vi "Autonomus.vi"(11 "RobotData":T1) -> ()   [LabVIEW 2019, in "Robot.lvlib" / "Panzer.lvclass"]
uses:
  Panzer.lvclass
  TypeDefs/RobotObjects.ctl
  Drive/Tank Drive/Tank Drive.lvclass
  Pnematics control/Pneumatics.lvclass
  Vision/Vision.lvclass
  Joysticks/Joysticks.lvclass
  Elevator/Elevator.lvclass
  Hatch/Hatch.lvclass
  Cargo/Cargo.lvclass
  DriveOld/Drive.lvclass
  Robot.lvclass
  Control Panel/Control Panel.lvclass
  Climber/Climber.lvclass
  Turret/Turret.lvclass
  PowerCellHandler/Power Cell Handler.lvclass
  Robot.lvclass/Robot.ctl
  PowerCellHandler/Controls/Shooting Position.ctl
  Data Members/Read Waits.vi
  Pnematics control/Solenoids/Solenoids.lvclass
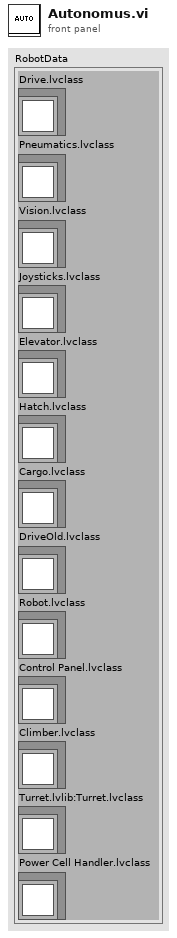
[diagram p1: front panel]
types:
  T1 = typedef "RobotObjects.ctl" = cluster{"Drive.lvclass":refnum<class "Tank Drive.lvclass">, "Pneumatics.lvclass":refnum<class "Pneumatics.lvclass">, "Vision.lvclass":refnum<class "Vision.lvclass">, "Joysticks.lvclass":refnum<class "Joysticks.lvclass">, "Elevator.lvclass":refnum<class "Elevator.lvclass">, "Hatch.lvclass":refnum<class "Hatch.lvclass">, "Cargo.lvclass":refnum<class "Cargo.lvclass">, "DriveOld.lvclass":refnum<class "Drive.lvclass">, "Robot.lvclass":refnum<class "Robot.lvclass">, "Control Panel.lvclass":refnum<class "Control Panel.lvclass">, "Climber.lvclass":refnum<class "Climber.lvclass">, "Turret.lvlib:Turret.lvclass":refnum<class "Turret.lvclass">, "Power Cell Handler.lvclass":refnum<class "Power Cell Handler.lvclass">}
  T2 = cluster{"Wait Before Shoot":dbl, "Wait Before Drive":dbl}
  T3 = typedef "Power Cell Handler.lvlib/Power Cell Handler.lvclass/Shooting Position.ctl" = enum16{"Rest", "Front", "Middle", "Back"}
  T4 = typedef "Pneumatics control.lvlib/Pneumatics.lvclass/Solenoids.ctl" = cluster{"Air Cooler":refnum<class "Solenoids.lvclass">, "ArmLock":refnum<class "Solenoids.lvclass">, "HatchArm":refnum<class "Solenoids.lvclass">, "HatchGrabber":refnum<class "Solenoids.lvclass">, "CPDeploy":refnum<class "Solenoids.lvclass">, "Power Cells Intake":refnum<class "Solenoids.lvclass">}
  T5 = typedef "Turret.lvlib/Turret.lvclass/Turret control states.ctl" = enum16{"Position", "Offset", "IMU"}
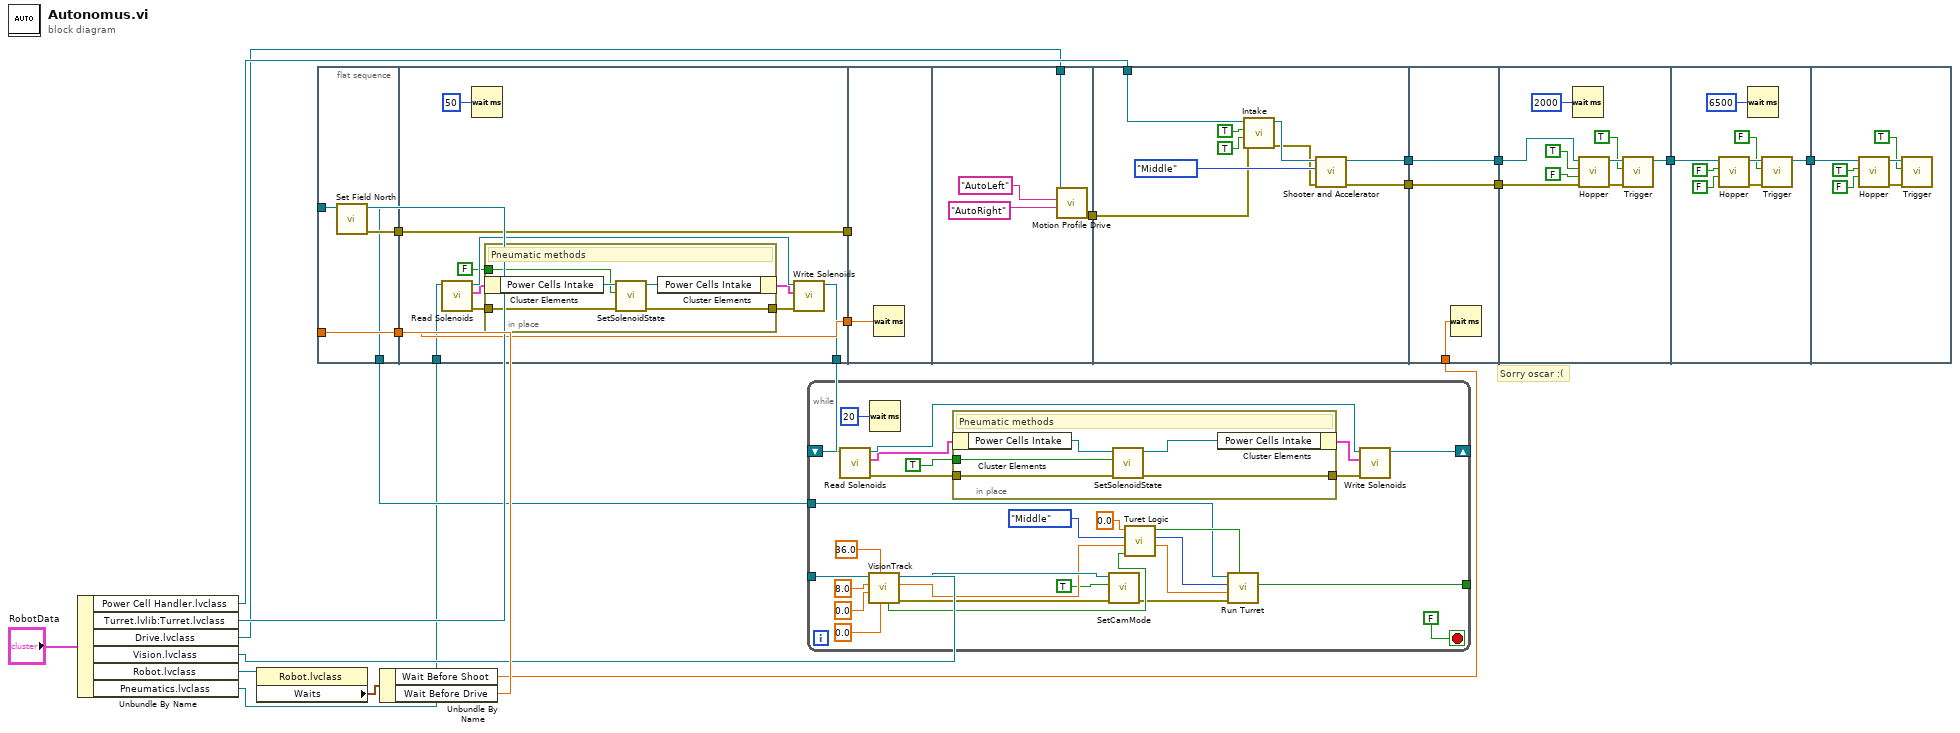
[diagram p0: block diagram]
diagram:
  # "Sorry oscar :("
  n1 = Unbundle By Name("RobotData") -> ("Power Cell Handler.lvclass"=w15:refnum<class "Power Cell Handler.lvclass">, "Turret.lvlib:Turret.lvclass"=w19:refnum<class "Turret.lvclass">, "Drive.lvclass"=w2:refnum<class "Tank Drive.lvclass">, "Vision.lvclass"=w17:refnum<class "Vision.lvclass">, "Robot.lvclass"=w22:refnum<class "Robot.lvclass">, "Pneumatics.lvclass"=w6:refnum<class "Pneumatics.lvclass">)
  n2 = property class="Robot.lvclass"(reference=w22) -> ("Waits"=w21:T2)  [unwired: 1 in, 2 out]
  n3 = flat-sequence {
    tunnel: w20 -> [w27]
    tunnel: [w25] -> w10
    tunnel: [w27] -> w8
    tunnel: w19 -> [w26]
    tunnel: [w24] -> w16
    tunnel: w10 -> [w38]
    tunnel: [w38] -> w9
    tunnel: w8 -> [w37]
    tunnel: [w37] -> w7
    tunnel: w6 -> [w29]
    tunnel: [w28] -> w5
    tunnel: w9 -> [_]
    tunnel: w7 -> [w44]
    tunnel: w2 -> [w46]
    tunnel: [w45] -> w1
    tunnel: w15 -> [w53]
    tunnel: [w56] -> w13
    tunnel: [w55] -> w12
    tunnel: w1 -> [w50]
    tunnel: w18 -> [w60]
    tunnel: [w59] -> w14
    tunnel: w13 -> [w59]
    tunnel: w12 -> [w58]
    tunnel: [w58] -> w11
    tunnel: w14 -> [w66]
    tunnel: w11 -> [w65]
    tunnel: [w61] -> w4
    tunnel: w4 -> [w72]
    tunnel: [w70] -> w3
    tunnel: w3 -> [w78]
    frame #0 {
      n4 = call "Set Field North.vi"("Turret in"=w26) -> ("error out"=w25:errorcluster, "Turret out"=w24:refnum<class "Turret.lvclass">)  [unwired: 9 in]
    }
    frame #1 {
      n5 = call-dynamic "Read Solenoids.vi"("Pneumatics in"=w29) -> ("error out"=w34:errorcluster, "Solenoids"=w35:T4, "Pneumatics out"=w36:refnum<class "Pneumatics.lvclass">)  [unwired: 8 in]
      n6 = Wait (ms)(milliseconds to wait=u32 50) -> ()  [unwired: 1 out]
      n7 = in-place {
        in-place-border: w34 -> [w42]
        in-place-border: [w40] -> w32
        in-place-border: FALSE ("f") -> [w39]
        # "Pneumatic methods"
        n8 = in-place-cluster #1(w35) -> ("Power Cells Intake"=w41:refnum<class "Solenoids.lvclass">)
        n9 = call-dynamic "SetSolenoidState.vi"("error in (no error)"=w42, "Solenoid On?"=w39, "Solenoids in"=w41) -> ("error out"=w40:errorcluster, "Solenoids out"=w43:refnum<class "Solenoids.lvclass">)  [unwired: 7 in]
        n10 = in-place-cluster #1("Power Cells Intake"=w43) -> (w33:T4)
      }
      n11 = call-dynamic "Write Solenoids.vi"("error in (no error)"=w32, "Solenoids"=w33, "Pneumatics in"=w36) -> ("Pneumatics out"=w28:refnum<class "Pneumatics.lvclass">)  [unwired: 7 in, 1 out]
    }
    frame #2 {
      n12 = Wait (ms)(milliseconds to wait=w44) -> ()  [unwired: 1 out]
    }
    frame #3 {
      n13 = call-dynamic "Motion Profile Drive.vi"("Right Buffer name"="AutoRight" ("Buffer Name"), "Left Buffer name"="AutoLeft" ("Buffer Name"), "Tank Drive in"=w46) -> ("error out"=w45:errorcluster)  [unwired: 7 in, 1 out]
    }
    frame #4 {
      n14 = call "Intake.vi"("error in (no error)"=w50, "Intake Running?"=TRUE, "Intake Out?"=TRUE, "Power Cell Handler in"=w53) -> ("error out"=w49:errorcluster, "Power Cell Handler out"=w54:refnum<class "Power Cell Handler.lvclass">)  [unwired: 5 in, 1 out]
      n15 = call "Shooter and Accelerator.vi"("error in (no error)"=w49, "Shooting Position"=Shooting_Position."Middle", "Power Cell Handler in"=w54) -> ("error out"=w55:errorcluster, "Power Cell Handler out"=w56:refnum<class "Power Cell Handler.lvclass">)  [unwired: 6 in, 1 out]
    }
    frame #5 {
      n16 = Wait (ms)(milliseconds to wait=w60) -> ()  [unwired: 1 out]
    }
    frame #6 {
      n17 = Wait (ms)(milliseconds to wait=u32 2000) -> ()  [unwired: 1 out]
      n18 = call "Hopper.vi"("error in (no error)"=w65, "Un Jam Mode"=FALSE, "Shooting"=TRUE, "Power Cell Handler in"=w66) -> ("error out"=w69:errorcluster, "Power Cell Handler out"=w68:refnum<class "Power Cell Handler.lvclass">)  [unwired: 6 in]
      n19 = call "Trigger.vi"("error in (no error)"=w69, "Shooting"=TRUE, "Power Cell Handler in"=w68) -> ("Power Cell Handler out"=w61:refnum<class "Power Cell Handler.lvclass">)  [unwired: 7 in, 1 out]
    }
    frame #7 {
      n20 = call "Hopper.vi"("Un Jam Mode"=FALSE, "Shooting"=FALSE, "Power Cell Handler in"=w72) -> ("error out"=w77:errorcluster, "Power Cell Handler out"=w76:refnum<class "Power Cell Handler.lvclass">)  [unwired: 7 in]
      n21 = Wait (ms)(milliseconds to wait=u32 6500) -> ()  [unwired: 1 out]
      n22 = call "Trigger.vi"("error in (no error)"=w77, "Shooting"=FALSE, "Power Cell Handler in"=w76) -> ("Power Cell Handler out"=w70:refnum<class "Power Cell Handler.lvclass">)  [unwired: 7 in, 1 out]
    }
    frame #8 {
      n23 = call "Hopper.vi"("Un Jam Mode"=FALSE, "Shooting"=TRUE, "Power Cell Handler in"=w78) -> ("error out"=w83:errorcluster, "Power Cell Handler out"=w82:refnum<class "Power Cell Handler.lvclass">)  [unwired: 7 in]
      n24 = call "Trigger.vi"("error in (no error)"=w83, "Shooting"=TRUE, "Power Cell Handler in"=w82) -> ()  [unwired: 7 in, 2 out]
    }
  }
  n25 = Unbundle By Name(w21) -> ("Wait Before Shoot"=w18:dbl, "Wait Before Drive"=w20:dbl)
  n26 = while {
    tunnel: w17 -> [w97]
    tunnel: w16 -> [w94]
    tunnel: [w93] -> _
    shift-right: [w85] -> _
    shift-left: w5 -> [w86]
    stop <- FALSE stop-if-true
    n27 = call-dynamic "Read Solenoids.vi"("Pneumatics in"=w86) -> ("error out"=w89:errorcluster, "Solenoids"=w90:T4, "Pneumatics out"=w91:refnum<class "Pneumatics.lvclass">)  [unwired: 8 in]
    n28 = call "VisionTrack.vi"("RobotLength (in)"=0.0, "target height(in)"=36.0, "mounting angle (degrees)"=0.0, "camera height(in)"=8.0, "Vision in"=w97) -> ("error out"=w105:errorcluster, "HorizontalOffset(degrees)"=w102:dbl, "Vision out"=w106:refnum<class "Vision.lvclass">, "Target?"=w104:bool)  [unwired: 1 in, 2 out]
    n29 = Wait (ms)(milliseconds to wait=u32 20) -> ()  [unwired: 1 out]
    n30 = in-place {
      in-place-border: w89 -> [w115]
      in-place-border: [w113] -> w87
      in-place-border: TRUE ("f") -> [w112]
      # "Pneumatic methods"
      n31 = in-place-cluster #2(w90) -> ("Power Cells Intake"=w114:refnum<class "Solenoids.lvclass">)
      n32 = call-dynamic "SetSolenoidState.vi"("error in (no error)"=w115, "Solenoid On?"=w112, "Solenoids in"=w114) -> ("error out"=w113:errorcluster, "Solenoids out"=w116:refnum<class "Solenoids.lvclass">)  [unwired: 7 in]
      n33 = in-place-cluster #2("Power Cells Intake"=w116) -> (w88:T4)
    }
    n34 = call "SetCamMode.vi"("Vision.lvlib:Vision.lvclass"=w106, "Vision Processing?"=TRUE, "error in (no error)"=w105) -> ("error out"=w103:errorcluster)  [unwired: 6 in, 1 out]
    n35 = call "Turet Logic.vi"("Vision Target?"=w104, "Vision Xoffset"=w102, "Shooting Position"=Shooting_Position."Middle", "Driver Xoffset"=0.0) -> ("Turret Offset(degrees)"=w109:dbl, "Turret mode"=w108:T5, "Scan Mode"=w107:bool)  [unwired: 4 in, 1 out]
    n36 = call "Run Turret.vi"("Search?"=w107, "error in (no error)"=w103, "Input(deg)"=w109, "Control mode"=w108, "Turret in"=w94) -> ("In Range?"=w93:bool)  [unwired: 4 in, 2 out]
    n37 = call-dynamic "Write Solenoids.vi"("error in (no error)"=w87, "Solenoids"=w88, "Pneumatics in"=w91) -> ("Pneumatics out"=w85:refnum<class "Pneumatics.lvclass">)  [unwired: 7 in, 1 out]
  }
